vi "GE5565 DMA Read Interrupt (U64) Cluster.vi"(6 "timeout (1000 ms)":u32=1000, 8 "error in (no error)":errorcluster, 10 "RM offset (0)":u32, 11 "VMIC reference in":T1) -> (0 "error out":errorcluster, 2 "buffer":dbl[](array[numeric]), 3 "VMIC reference out":T1)   [LabVIEW 2015, in "RefMem DMA Custom Device.lvlib"]
uses:
  <vilib>/Instr/_visa.llb/Select Event Type.ctl
  RefMem DMA Custom Device.lvlib
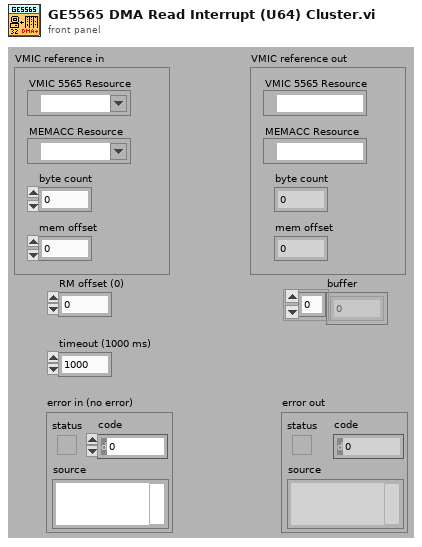
[diagram p1: front panel]
types:
  T1 = cluster{"VMIC 5565 Resource":refnum<visa-resource-name>, "MEMACC Resource":refnum<visa-resource-name>, "byte count":u32, "mem offset":u32}
  T2 = typedef "Select Event Type.ctl" = u32
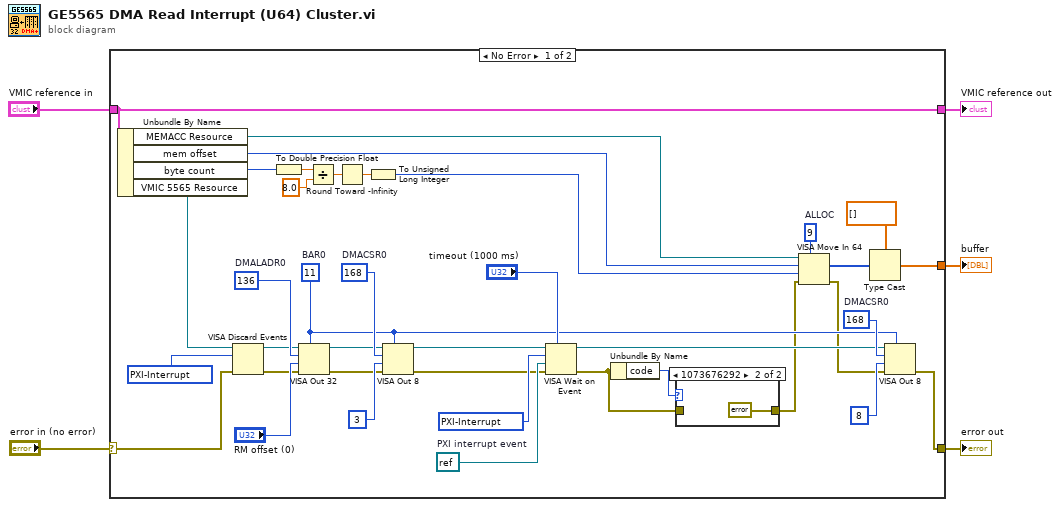
[diagram p0: block diagram]
diagram:
  n1 = case shown="No Error" "error in (no error)" {
    selector: "error in (no error)" -> [w32 w46]
    tunnel: "VMIC reference in" -> [w22 w47]
    tunnel: [w22 w47] -> w2
    tunnel: [w12 w46] -> w4
    tunnel: [w9 _] -> w1
    frame No Error {
      w37 = u16 9  # ALLOC
      w14 = u16 11  # BAR0
      w34 = refnum<visa-resource-name> refnum  # PXI interrupt event
      w17 = u32 168  # DMACSR0
      w29 = T2 1073684514 items=["ServiceRequest"=1073684491, "Trigger"=3221168138, "Clear"=1073684493, "VXI-Signal"=1073684512, "VXI/VME-Interrupt"=3221168161, "VXI/VME-Sysfail"=1073684509, "VXI/VME-Sysreset"=1073684510, "GPIB-CIC"=1073684498, "GPIB-Talk"=1073684499, "GPIB-Listen"=1073684500, "PXI-Interrupt"=1073684514, "AllEnabled"=1073709055] ("Event Type")
      w35 = T2 1073684514 items=["ServiceRequest"=1073684491, "Trigger"=3221168138, "Clear"=1073684493, "VXI-Signal"=1073684512, "VXI/VME-Interrupt"=3221168161, "VXI/VME-Sysfail"=1073684509, "VXI/VME-Sysreset"=1073684510, "GPIB-CIC"=1073684498, "GPIB-Talk"=1073684499, "GPIB-Listen"=1073684500, "PXI-Interrupt"=1073684514, "AllEnabled"=1073709055] ("Event Type")
      w42 = u32 168  # DMACSR0
      w43 = u32 136  # DMALADR0
      n2 = Unbundle By Name(w22) -> ("MEMACC Resource"=w19:refnum<visa-resource-name>, "mem offset"=w20:u32, "byte count"=w21:u32, "VMIC 5565 Resource"=w23:refnum<visa-resource-name>)
      n3 = VISA Discard Events(8:w32, 10:w29, 11:w23) -> (0:w30:errorcluster, 3:w31:refnum<visa-resource-name>)  [unwired: 1 in]
      n4 = To Double Precision Float(number=w21) -> (double precision float=w28:dbl)
      n5 = VISA Out 32(7:w14, 8:w30, 9:"RM offset (0)", 10:w43, 11:w31) -> (0:w39:errorcluster, 3:w40:refnum<visa-resource-name>)
      n6 = Divide(x=w28, y=8.0) -> (x/y=w26:dbl)
      n7 = Round Toward -Infinity(1:w26) -> (0:w25:dbl)
      n8 = To Unsigned Long Integer(number=w25) -> (unsigned 32bit integer=w24:u32)
      n9 = VISA Out 8(7:w14, 8:w39, 9:u8 3 ("value (0)"), 10:w42, 11:w40) -> (0:w18:errorcluster, 3:w33:refnum<visa-resource-name>)
      n10 = VISA Wait on Event(7:"timeout (1000 ms)", 8:w18, 9:w34, 10:w35, 11:w33) -> (0:w8:errorcluster, 3:w15:refnum<visa-resource-name>)  [unwired: 2 out]
      n11 = Unbundle By Name(w8) -> ("code"=w6:i32)
      n12 = case shown="1073676292" w6 {
        tunnel: [w44 errorcluster {"status"=FALSE, "code"=0, "source"=""} ("error out")] -> w7
        tunnel: w8 -> [w44 _]
        frame 0, Default {
        }
        frame 1073676292 {
        }
      }
      n13 = VISA Move In 64(7:w37, 8:w7, 9:w24, 10:w20, 11:w19) -> (0:w13:errorcluster, 2:w11:u64[])  [unwired: 1 out]
      n14 = Type Cast(type=dbl[] [] ("buffer"), x=w11) -> (*(type *) &x=w9:dbl[])
      n15 = VISA Out 8(7:w14, 8:w13, 9:u8 8 ("value (0)"), 10:w17, 11:w15) -> (0:w12:errorcluster)  [unwired: 1 out]
    }
    frame Error {
    }
  }
  "error out" <- w4
  "VMIC reference out" <- w2
  "buffer" <- w1
